vi "Generate Sequence.vi"(8 "error in (no error)":errorcluster, 11 "Toggle 7.1 in":refnum<class "Toggle 7.1.lvclass">) -> (0 "error out":errorcluster, 3 "Toggle 7.1 out":refnum<class "Toggle 7.1.lvclass">)   [LabVIEW 2020, in "Toggle 7.1.lvclass"]
doc: "Generates the test sequence and puts this into the class data"
uses:
  Toggle 7.1.lvclass
  C:/Sandbox/Git_Sandbox/WiSpry Test Framework source code (LV20)/WiSpry Test Framework/Devices/Device.lvclass
  Controls/Test Sequence.ctl
  Controls/Register to Write.ctl
  Controls/EFuse modes enum.ctl
  PIC-device/PIC-Device.lvclass
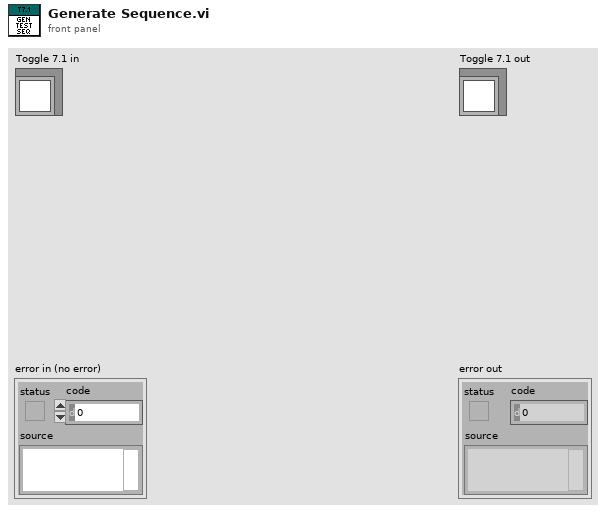
[diagram p1: front panel]
types:
  T1 = typedef "Toggle 7.1.lvclass/Test Sequence.ctl" = cluster{"Charge Pump Settings":T2[], "Charge Pump Values":dbl[], "Efuse Register Array":T2[], "Efuse Array":T3[], "Cap Register Array":T2[], "Cap Value Array":cluster{"Register Number":u32, "Value":dbl}[], "DWA Settings":T2[], "DWA Values":dbl[]}
  T2 = typedef "PIC-Device.lvclass/Register to Write.ctl" = cluster{"Register":u32, "Value":u32, "Dev Address":u32, "Physical Adress":u32}
  T3 = typedef "Toggle 7.1.lvclass/EFuse modes enum.ctl" = enum16{"On", "Off", "Both On and Off"}
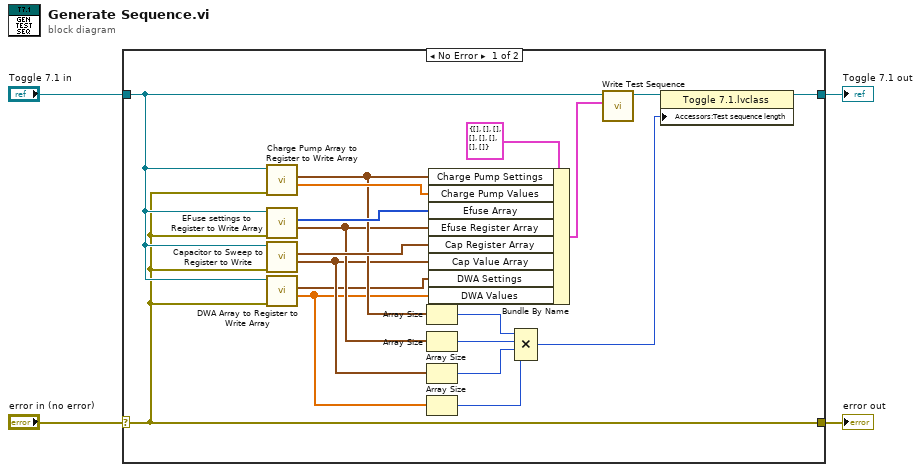
[diagram p0: block diagram]
diagram:
  n1 = case shown="No Error" "error in (no error)" {
    selector: "error in (no error)" -> [w11 w25]
    tunnel: [w11 w25] -> w3
    tunnel: [w6 w24] -> w1
    tunnel: "Toggle 7.1 in" -> [w12 w24]
    frame No Error {
      n2 = call "Charge Pump Array to Register to Write Array.vi"("error in (no error)"=w11, "Toggle 6 in"=w12) -> ("Charge Pump Values"=w23:dbl[], "Charge Pump Settings"=w18:T2[])  [unwired: 6 in, 2 out]
      n3 = call "EFuse settings to Register to Write Array.vi"("error in (no error)"=w11, "Toggle 6 in"=w12) -> ("Efuse Register Array"=w17:T2[], "Efuse Array"=w22:T3[])  [unwired: 6 in, 2 out]
      n4 = call "Capacitor to Sweep to Register to Write.vi"("error in (no error)"=w11, "Toggle 7.1 in"=w12) -> ("Cap Value Array"=w16:cluster{"Register Number":u32, "Value":dbl}[], "Cap Register Array"=w21:T2[])  [unwired: 6 in, 2 out]
      n5 = call "DWA Array to Register to Write Array.vi"("error in (no error)"=w11, "Toggle 7.1 in"=w12) -> ("DWA Values"=w9:dbl[], "DWA Settings"=w10:T2[])  [unwired: 6 in, 2 out]
      n6 = Array Size(array=w18) -> (size(s)=w15:i32)
      n7 = Array Size(array=w17) -> (size(s)=w14:i32)
      n8 = Array Size(array=w16) -> (size(s)=w13:i32)
      n9 = Array Size(array=w9) -> (size(s)=w8:i32)
      n10 = Bundle By Name(cluster=T1 {"Charge Pump Settings"=[], "Charge Pump Values"=[], "Efuse Register Array"=[], "Efuse Array"=[], "Cap Register Array"=[], "Cap Value Array"=[], "DWA Settings"=[], "DWA Values"=[]}, "Charge Pump Settings"=w18, "Charge Pump Values"=w23, "Efuse Array"=w22, "Efuse Register Array"=w17, "Cap Register Array"=w21, "Cap Value Array"=w16, "DWA Settings"=w10, "DWA Values"=w9) -> (w19:T1)
      n11 = Compound Arithmetic op=MULTIPLY(w15, w14, w13, w8) -> (w5:i32)
      n12 = call-dynamic "Write Test Sequence.vi"("Test Sequence"=w19, "Toggle 6 in"=w12) -> ("Toggle 6 out"=w7:refnum<class "Toggle 7.1.lvclass">)  [unwired: 9 in]
      n13 = property class="Toggle 7.1.lvclass"(reference=w7, "Accessors:Test sequence length"=w5) -> (reference out=w6:refnum<class "Toggle 7.1.lvclass">)  [unwired: 1 in, 1 out]
    }
    frame Error {
    }
  }
  "error out" <- w3
  "Toggle 7.1 out" <- w1
